vi "New.vi"() -> (3 "Signaller out":refnum<class "Signaller.lvclass">)   [LabVIEW 2015, in "Signaller.lvclass"]
uses:
  Signaller.lvclass
  Signaller.lvclass/Signaller.ctl
panel:
  out "Error out":errorcluster
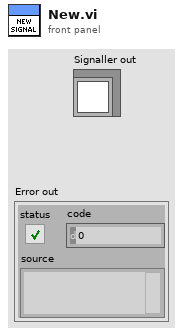
[diagram p1: front panel]
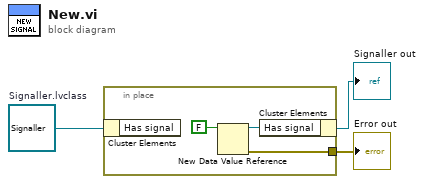
[diagram p0: block diagram]
diagram:
  w3 = refnum<class "Signaller.lvclass"> refnum  # Signaller.lvclass
  n1 = in-place {
    in-place-border: [w4] -> w1
    n2 = in-place-cluster #1(w3) -> ()  [unwired: 1 out]
    n3 = New Data Value Reference(data value=FALSE) -> (data value reference=w5:refnum<data-value>, error out=w4:errorcluster)  [unwired: 1 in]
    n4 = in-place-cluster #1("Has signal"=w5) -> (→"Signaller out":refnum<class "Signaller.lvclass">)
  }
  "Error out" <- w1
